vi "Memory.Pointer.Errors.Get Info.vi"(11 "error":T1) -> (3 "error info":cluster{"code":i32, "description":string})   [LabVIEW 2016, in "Memory.lvlib" / "Memory.Pointer.lvclass"]
uses:
  Memory.Pointer.lvclass
  Memory.Pointer.Errors.ctl
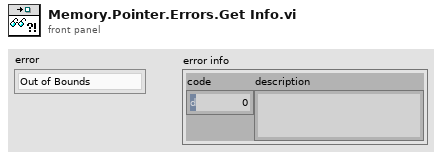
[diagram p1: front panel]
types:
  T1 = typedef "Memory.lvlib/Memory.Pointer.lvclass/Memory.Pointer.Errors.ctl" = enum16{"Out of Bounds", "Buffer Underflow", "Size Mismatch", "Zone", "Null Pointer"}
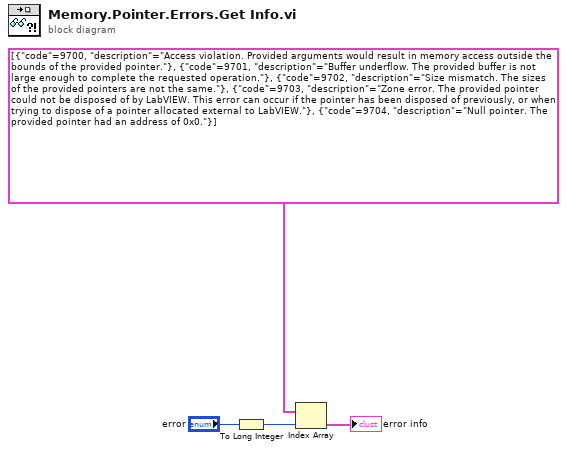
[diagram p0: block diagram]
diagram:
  n1 = To Long Integer(number="error") -> (32bit integer=w3:i32)
  n2 = Index Array(array=cluster{"code":i32, "description":string}[] [{"code"=9700, "description"="Access violation. Provided arguments would result in memory access outside the bounds of the provided pointer."}, {"code"=9701, "description"="Buffer underflow. The provided buffer is not large enough to complete the requested operation."}, {"code"=9702, "description"="Size mismatch. The sizes of the provided pointers are not the same."}, {"code"=9703, "description"="Zone error. The provided pointer could not be disposed of by LabVIEW. This error can occur if the pointer has been disposed of previously, or when trying to dispose of a pointer allocated external to LabVIEW."}, {"code"=9704, "description"="Null pointer. The provided pointer had an address of 0x0."}] ("error info"), index=w3) -> (element=→"error info":cluster{"code":i32, "description":string})
